vi "CreateSingleVibrationTDMSFile.vi"(0 "Requested Directory":path, 1 "Device":T4, 2 "Hierarchy":T1, 5 "Number of Channels":i32=18, 7 "Tach?":bool=TRUE, 9 "Pairs?":bool=TRUE, 11 "All Accelerometers?":bool=TRUE, 12 "sampling info":cluster{"Fs":dbl, "#s":dbl}={"Fs"=10000.0, "#s"=100000.0} {"Fs" format="%.2p"}, 13 "Running Speed (RPM)":dbl=3600.0, 14 "Amplitude":T11={"1x"=1.0, "2x"=0.5, "3x"=0.25, "8.5x"=1.0, "30x"=1.0}) -> (4 "Created File":path, 15 "error out":errorcluster)   [LabVIEW 2017]
uses:
  <vilib>/addons/InsightCM/MessageBus/Base/controls/Device.ctl
  <vilib>/addons/InsightCM/MessageBus/Base/controls/KeyValuePair.ctl
  <vilib>/addons/InsightCM/MessageBus/Base/controls/DeviceState.ctl
  <vilib>/addons/InsightCM/MessageBus/Base/controls/DataGroup.ctl
  <vilib>/addons/InsightCM/MessageBus/Base/controls/BurstModeTrigger.ctl
  <vilib>/addons/InsightCM/MessageBus/Base/controls/Trigger.ctl
  <vilib>/addons/InsightCM/MessageBus/Base/controls/Condition.ctl
  <vilib>/addons/InsightCM/Utilities/TDMSFileGenerator/controls/Hierarchy_All.ctl
  <vilib>/addons/InsightCM/Utilities/TDMSFileGenerator/controls/Hierarchy_Line.ctl
  <vilib>/addons/InsightCM/Utilities/TDMSFileGenerator/controls/Hierarchy_Equipment.ctl
  <vilib>/measure/NI_MABase.lvlib
  <vilib>/addons/Sound and Vibration/svt_DAQmx/Configuration XControl/Controls/svx_DAQ_RotationDirection.ctl
  <vilib>/addons/Sound and Vibration/svt_DAQmx/Configuration XControl/SVX NI-DAQmx AI Configuration XControl.xctl
  <vilib>/addons/Sound and Vibration/svt_DAQmx/Configuration XControl/Controls/svx_DAQ_Tach_Slope.ctl
panel:
  out "Array":i32[](array[numeric])
  out "Channel Names":string[](array[string])
  out "Waveforms":waveform(sgl)[](graph)
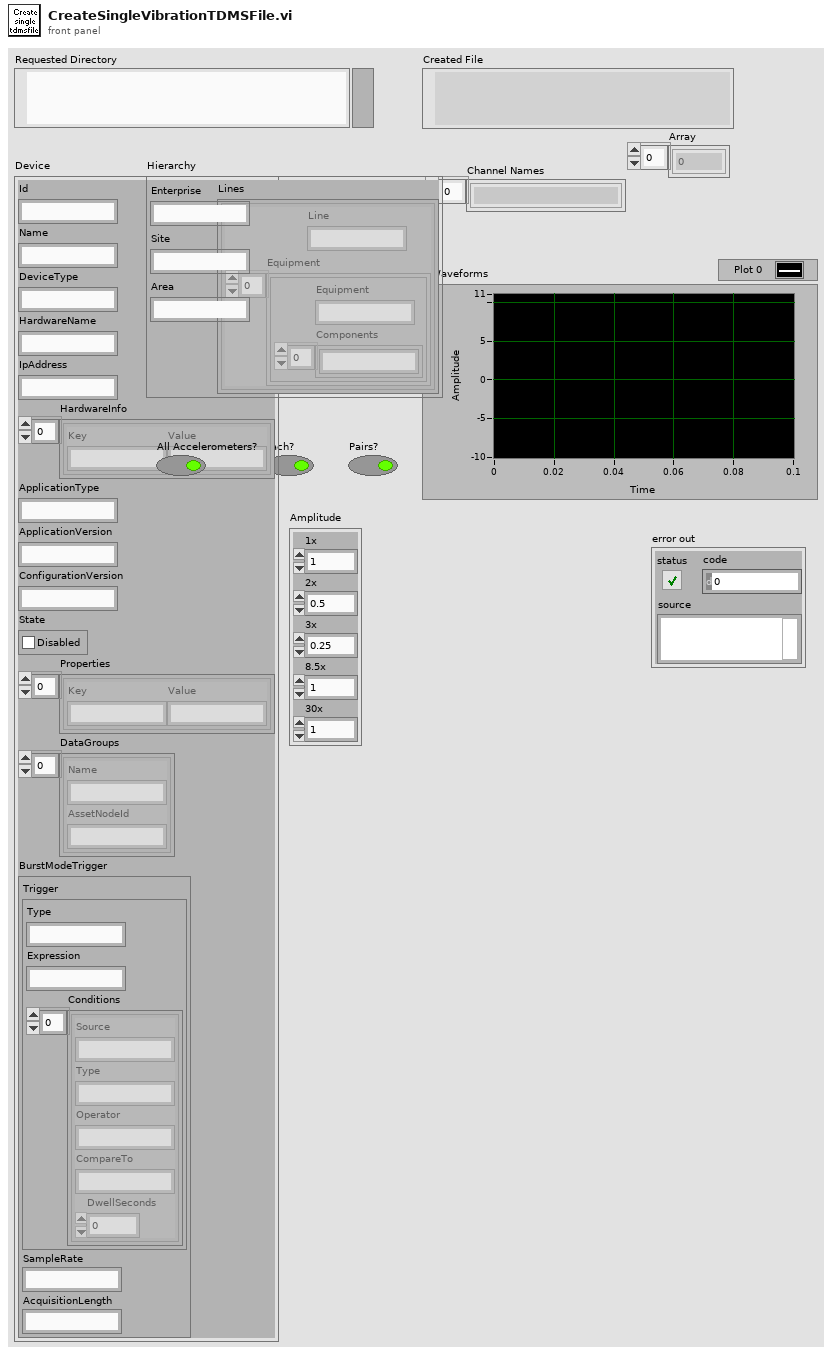
[diagram p1: front panel]
types:
  T1 = typedef "Hierarchy_All.ctl" = cluster{"Enterprise":string, "Site":string, "Area":string, "Lines":T2[]}
  T2 = typedef "Hierarchy_Line.ctl" = cluster{"Line":string, "Equipment":T3[]}
  T3 = typedef "Hierarchy_Equipment.ctl" = cluster{"Equipment":string, "Components":string[]}
  T4 = typedef "Device.ctl" = cluster{"Id":string, "Name":string, "DeviceType":string, "HardwareName":string, "IpAddress":string, "HardwareInfo":T5[], "ApplicationType":string, "ApplicationVersion":string, "ConfigurationVersion":string, "State":T6, "Properties":T5[], "DataGroups":T7[], "BurstModeTrigger":T8}
  T5 = typedef "KeyValuePair.ctl" = cluster{"Key":string, "Value":string}
  T6 = typedef "DeviceState.ctl" = cluster{"Disabled":bool}
  T7 = typedef "DataGroup.ctl" = cluster{"Name":string, "AssetNodeId":string}
  T8 = typedef "BurstModeTrigger.ctl" = cluster{"Trigger":T9, "SampleRate":string, "AcquisitionLength":string}
  T9 = typedef "Trigger.ctl" = cluster{"Type":string, "Expression":string, "Conditions":T10[]}
  T10 = typedef "Condition.ctl" = cluster{"Source":string, "Type":string, "Operator":string, "CompareTo":string, "DwellSeconds":dbl}
  T11 = cluster{"1x":dbl, "2x":dbl, "3x":dbl, "8.5x":dbl, "30x":dbl}
  T12 = enum16{"open", "open or create", "create or replace", "create", "open (read-only)"}
  T13 = typedef "SVX NI-DAQmx AI Configuration XControl.xctl/svx_DAQ_Tach_Slope.ctl" = enum16{"Rising", "Falling"}
  T14 = typedef "SVX NI-DAQmx AI Configuration XControl.xctl/svx_DAQ_RotationDirection.ctl" = enum16{"CW", "CCW"}
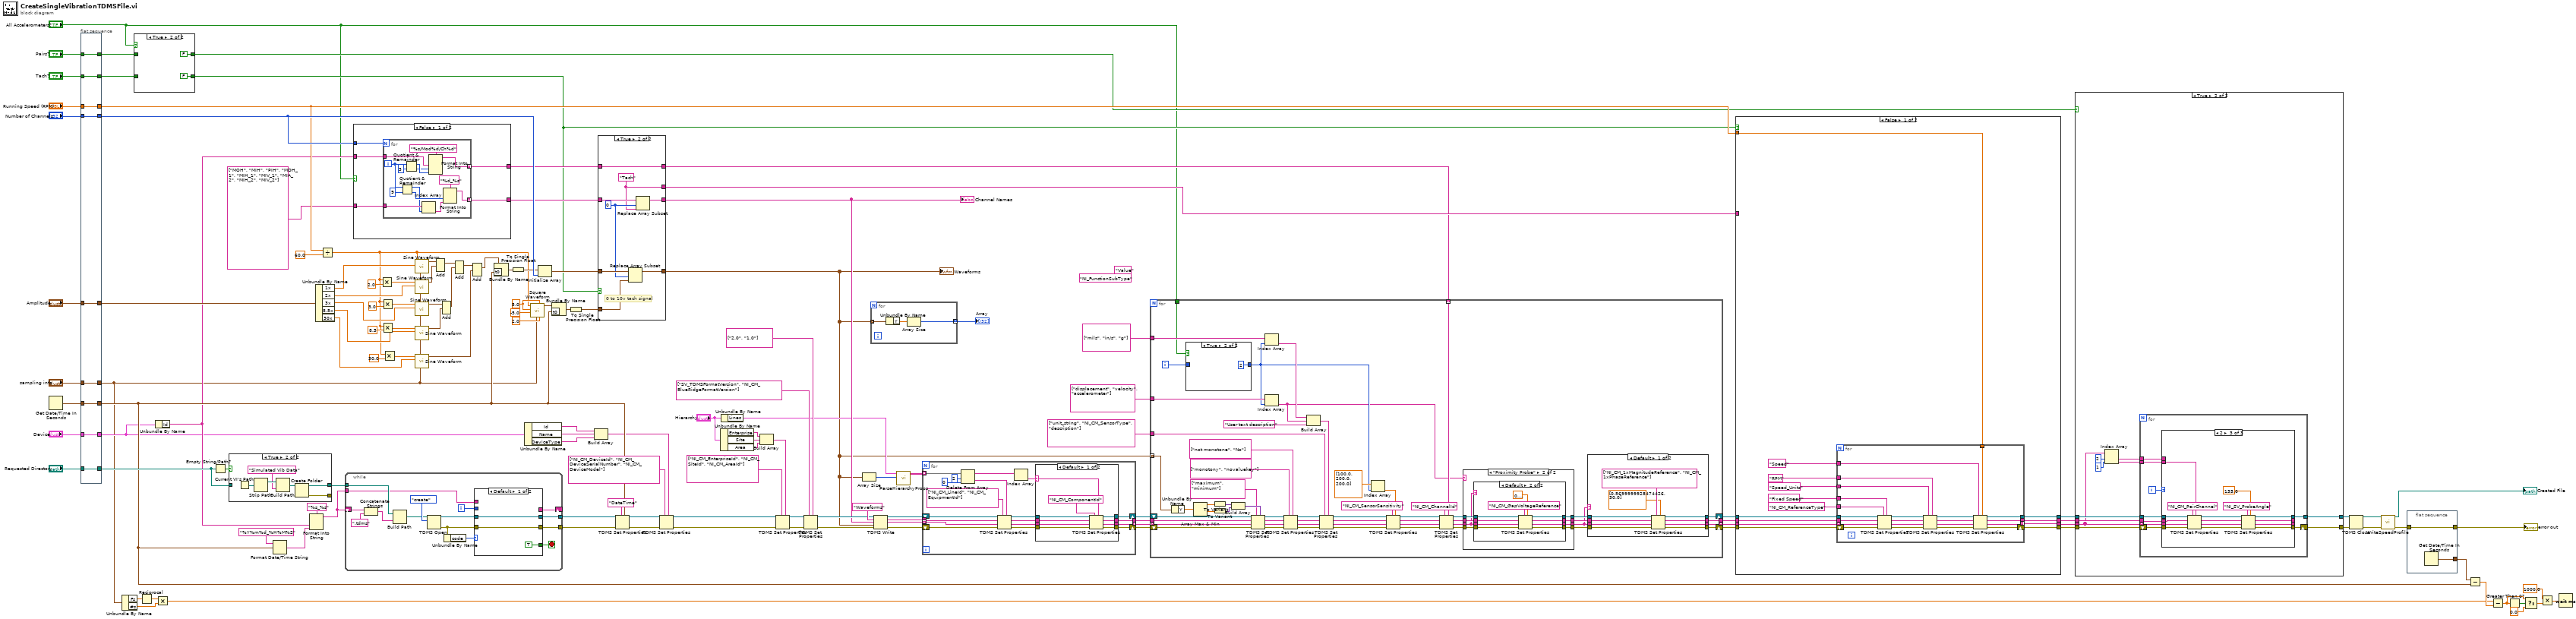
[diagram p0: block diagram]
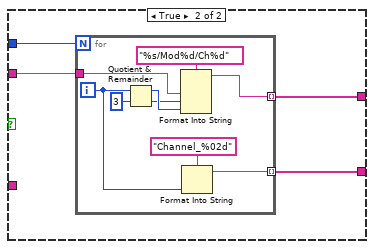
[diagram p2: hidden frame]
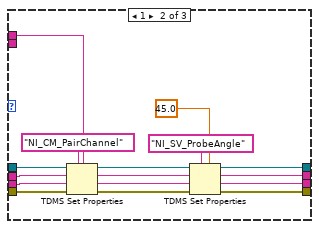
[diagram p7: hidden frame]
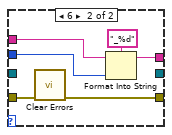
[diagram p8: hidden frame]
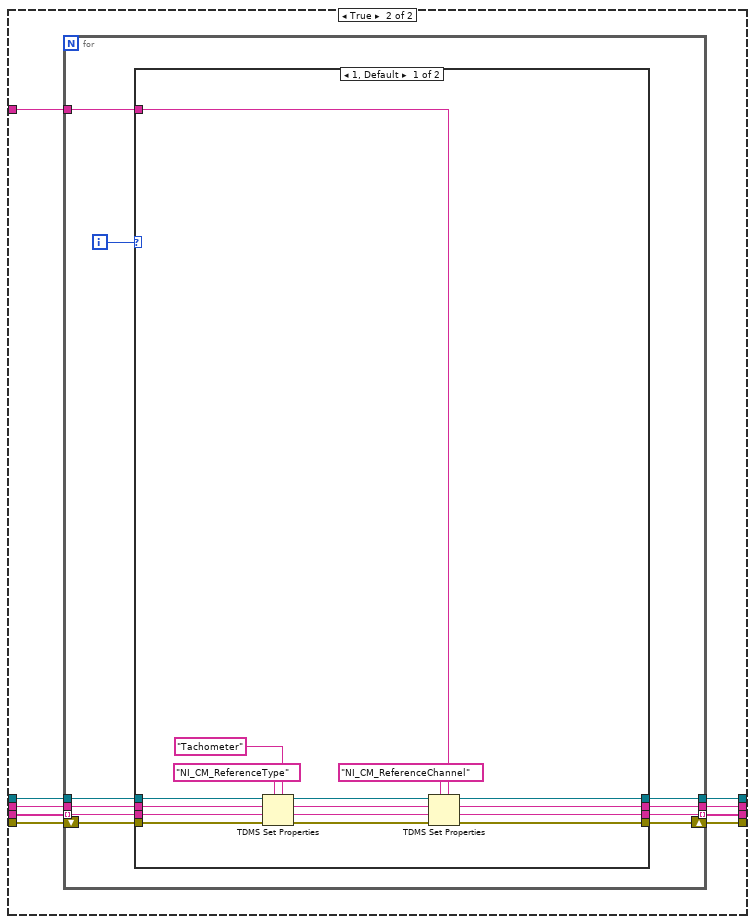
[diagram p10: hidden frame]
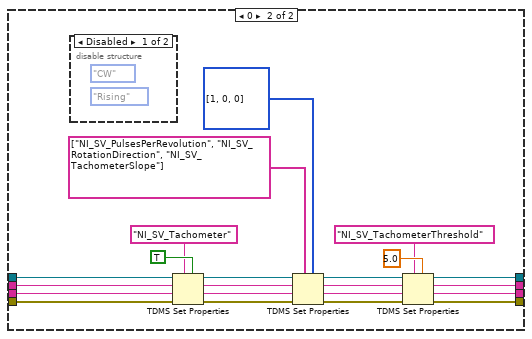
[diagram p11: hidden frame]
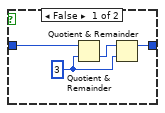
[diagram p13: hidden frame]
diagram:
  (unwired) "NI_FunctionSubType"
  w69 = 5.0 ("amplitude")
  (unwired) "Value"
  n1 = Get Date/Time In Seconds() -> (seconds since 1Jan1904=w92:timestamp)
  n2 = flat-sequence {
    tunnel: [w144] -> w101
    tunnel: "Requested Directory" -> [w144]
    tunnel: [w143] -> w11
    tunnel: "sampling info" -> [w143]
    tunnel: [w142] -> w98
    tunnel: "Amplitude" -> [w142]
    tunnel: [w141] -> w96
    tunnel: "Number of Channels" -> [w141]
    tunnel: [w140] -> w94
    tunnel: "Running Speed (RPM)" -> [w140]
    tunnel: [w139] -> w13
    tunnel: "Tach?" -> [w139]
    tunnel: [w138] -> w67
    tunnel: w92 -> [w138]
    tunnel: [w137] -> w15
    tunnel: "Pairs?" -> [w137]
    tunnel: "Device" -> [w136]
    tunnel: [w136] -> w43
    frame #0 {
    }
  }
  n3 = Unbundle By Name(w11) -> ("Fs"=w90:dbl, "#s"=w88:dbl)
  n4 = case shown="True" "All Accelerometers?" {
    tunnel: [w146 FALSE ("Pairs?")] -> w14
    tunnel: w15 -> [w146 _]
    tunnel: [w145 FALSE ("Tach?")] -> w12
    tunnel: w13 -> [w145 _]
    frame False {
    }
    frame True {
    }
  }
  n5 = Reciprocal(x=w90) -> (1/x=w89:dbl)
  n6 = Unbundle By Name(w43) -> ("Id"=w44:string)
  n7 = Multiply(x=w89, y=w88) -> (x*y=w86:dbl)
  n8 = Empty String/Path?(string/path=w101) -> (empty?=w121:bool)
  n9 = case shown="True" w121 {
    tunnel: [w149 w151] -> w122
    tunnel: w101 -> [w149 _]
    tunnel: [_ w150] -> _
    frame False {
    }
    frame True {
      n10 = Current VI's Path() -> (path=w155:path)
      n11 = Strip Path(path=w155) -> (stripped path=w154:path)  [unwired: 1 out]
      n12 = Build Path(base path=w154, name or relative path="Simulated Vib Data") -> (appended path=w152:path)
      n13 = Create Folder(path (use dialog)=w152) -> (created path=w151:path, error out=w150:errorcluster)  [unwired: 2 in, 1 out]
    }
  }
  n14 = Format Date/Time String(time format string (%c)="%Y%m%d_%H%M%S" ("format string"), seconds (now)=w67) -> (date/time string=w125:string)  [unwired: 1 in]
  n15 = Format Into String(format string="%s_%s", w44, w125) -> (resulting string=w103:string)  [unwired: 2 in, 1 out]
  n16 = Unbundle By Name(w98) -> ("1x"=w106:dbl, "2x"=w107:dbl, "3x"=w104:dbl, "8.5x"=w105:dbl, "30x"=w7:dbl)
  n17 = Divide(x=w94, y=60.0) -> (x/y=w8:dbl)
  n18 = while {
    tunnel: [w164] -> w132
    tunnel: [w166] -> w131
    tunnel: w122 -> [w168]
    shift-right: [w157] -> _
    shift-left: w103 -> [w161]
    tunnel: w103 -> [w159]
    i -> [w158]
    stop <- w167 stop-if-true
    n19 = Concatenate Strings(w161, ".tdms" ("format string")) -> (w160:string)
    n20 = Build Path(base path=w168, name or relative path=w160) -> (appended path=w169:path)
    n21 = TDMS Open(10:T12."create" ("operation (0:open)"), 11:w169) -> (0:w162:errorcluster, 3:w165:refnum<k34>)  [unwired: 5 in]
    n22 = Unbundle By Name(w162) -> ("code"=w163:i32)
    n23 = case shown="Default" w163 {
      tunnel: [TRUE _] -> w167
      tunnel: [w172 _] -> w166
      tunnel: w165 -> [w172 _]
      tunnel: [w171 w178] -> w164
      tunnel: w162 -> [w171 w179]
      tunnel: w159 -> [_ w177]
      tunnel: w158 -> [_ w175]
      tunnel: [_ w174] -> w157
      frame Default {
      }
      frame 6 {
        n24 = call <vilib>:"Clear Errors.vi"("error in (no error)"=w179) -> ("error out"=w178:errorcluster)  [unwired: 5 in, 1 out]
        n25 = Format Into String(format string="_%d", initial string=w177, w175) -> (resulting string=w174:string)  [unwired: 1 in, 1 out]
      }
    }
  }
  n26 = case shown="False" "All Accelerometers?" {
    tunnel: w96 -> [w184 w202]
    tunnel: string[] ["MOH", "MIH", "PIH", "MOH_1", "MIH_1", "MIV_1", "MIA_2", "MIH_2", "MIV_2"] ("property names") -> [w183 _]
    tunnel: [w182 w201] -> w60
    tunnel: [w181 w200] -> w59
    tunnel: w44 -> [w180 w199]
    frame False {
      n27 = for {
        N: w184 -> [_]
        tunnel: [w198] -> w181 mode=indexing
        tunnel: w180 -> [w197]
        tunnel: w183 -> [w187]
        tunnel: [w189] -> w182 mode=indexing
        i -> [w192]
        n28 = Quotient & Remainder(x=w192, y=9) -> (x-y*floor(x/y)=w185:i32, floor(x/y)=w188:i32)
        n29 = Quotient & Remainder(x=w192, y=3) -> (x-y*floor(x/y)=w195:i32, floor(x/y)=w194:i32)
        n30 = Index Array(array=w187, index=w185) -> (element=w186:string)
        n31 = Format Into String(format string="%s/Mod%d/Ch%d", w197, w194, w195) -> (resulting string=w198:string)  [unwired: 2 in, 1 out]
        n32 = Format Into String(format string="%d_%s", w188, w186) -> (resulting string=w189:string)  [unwired: 2 in, 1 out]
      }
    }
    frame True {
      n33 = for {
        N: w202 -> [_]
        tunnel: [w211] -> w200 mode=indexing
        tunnel: w199 -> [w210]
        tunnel: [w203] -> w201 mode=indexing
        i -> [w204]
        n34 = Quotient & Remainder(x=w204, y=3) -> (x-y*floor(x/y)=w208:i32, floor(x/y)=w207:i32)
        n35 = Format Into String(format string="%s/Mod%d/Ch%d", w210, w207, w208) -> (resulting string=w211:string)  [unwired: 2 in, 1 out]
        n36 = Format Into String(format string="Channel_%02d", w204) -> (resulting string=w203:string)  [unwired: 2 in, 1 out]
      }
    }
  }
  n37 = Multiply(x=w8, y=2.0) -> (x*y=w120:dbl)
  n38 = Multiply(x=w8, y=3.0) -> (x*y=w116:dbl)
  n39 = Multiply(x=w8, y=8.5) -> (x*y=w115:dbl)
  n40 = Multiply(x=w8, y=30.0) -> (x*y=w9:dbl)
  n41 = call <vilib>:"Sine Waveform.vi"("sampling info"=w11, "amplitude"=w106, "frequency"=w8) -> ("signal out"=w114:waveform(dbl))  [unwired: 7 in, 1 out]
  n42 = call <vilib>:"Sine Waveform.vi"("sampling info"=w11, "amplitude"=w107, "frequency"=w120) -> ("signal out"=w113:waveform(dbl))  [unwired: 7 in, 1 out]
  n43 = call <vilib>:"Sine Waveform.vi"("sampling info"=w11, "amplitude"=w104, "frequency"=w116) -> ("signal out"=w112:waveform(dbl))  [unwired: 7 in, 1 out]
  n44 = call <vilib>:"Sine Waveform.vi"("sampling info"=w11, "amplitude"=w105, "frequency"=w115) -> ("signal out"=w111:waveform(dbl))  [unwired: 7 in, 1 out]
  n45 = call <vilib>:"Sine Waveform.vi"("sampling info"=w11, "amplitude"=w7, "frequency"=w9) -> ("signal out"=w5:waveform(dbl))  [unwired: 7 in, 1 out]
  n46 = Add(1:w113, 2:w114) -> (0:w110:waveform(dbl))  [unwired: 1 in, 1 out]
  n47 = Add(1:w111, 2:w112) -> (0:w109:waveform(dbl))  [unwired: 1 in, 1 out]
  n48 = Add(1:w109, 2:w110) -> (0:w6:waveform(dbl))  [unwired: 1 in, 1 out]
  n49 = Add(1:w5, 2:w6) -> (0:w4:waveform(dbl))  [unwired: 1 in, 1 out]
  n50 = Bundle By Name(cluster=w4, "t0"=w67) -> (w73:waveform(dbl))
  n51 = To Single Precision Float(number=w73) -> (single precision float=w72:waveform(sgl))
  n52 = Unbundle By Name(w43) -> ("Id"=w41:string, "Name"=w42:string, "DeviceType"=w40:string)
  n53 = call <vilib>:"Square Waveform.vi"("duty cycle (%)"=2.0, "offset"=w69, "sampling info"=w11, "phase"=-5.0, "amplitude"=w69, "frequency"=w8) -> ("signal out"=w71:waveform(dbl))  [unwired: 4 in, 1 out]
  n54 = Initialize Array(w72, w96) -> (w108:waveform(sgl)[])
  n55 = Bundle By Name(cluster=w71, "t0"=w67) -> (w66:waveform(dbl))
  n56 = To Single Precision Float(number=w66) -> (single precision float=w65:waveform(sgl))
  n57 = Build Array(w41, w42, w40) -> (w39:string[])
  n58 = case shown="True" w12 {
    tunnel: w108 -> [w214 w222]
    tunnel: [w214 w221] -> w2
    tunnel: w60 -> [w213 w219]
    tunnel: w65 -> [_ w220]
    tunnel: [w213 w218] -> w58
    tunnel: w59 -> [w212 w216]
    tunnel: [w212 w216] -> w56
    tunnel: [_ w215] -> w57
    frame False {
    }
    frame True {
      w215 = "Tach" ("new element/subarray")
      w217 = 0 ("index")
      # "0 to 10v tach signal"
      n59 = Replace Array Subset(array=w222, new element=w220, index=w217) -> (w221:waveform(sgl)[])
      n60 = Replace Array Subset(array=w219, new element=w215, index=w217) -> (w218:string[])
    }
  }
  "Waveforms" <- w2
  "Channel Names" <- w58
  n61 = TDMS Set Properties(5:w67, 7:"DateTime" ("property names"), 8:w132, 11:w131) -> (0:w128:errorcluster, 3:w127:refnum<k34>)  [unwired: 2 in, 2 out]
  n62 = TDMS Set Properties(5:w39, 7:string[] ["NI_CM_DeviceId", "NI_CM_DeviceSerialNumber", "NI_CM_DeviceModel"], 8:w128, 11:w127) -> (0:w37:errorcluster, 3:w38:refnum<k34>)  [unwired: 2 in, 2 out]
  n63 = Unbundle By Name("Hierarchy") -> ("Enterprise"=w32:string, "Site"=w33:string, "Area"=w31:string)
  n64 = Unbundle By Name("Hierarchy") -> ("Lines"=w28:T2[])
  n65 = Build Array(w32, w33, w31) -> (w30:string[])
  n66 = TDMS Set Properties(5:w30, 7:string[] ["NI_CM_EnterpriseId", "NI_CM_SiteId", "NI_CM_AreaId"], 8:w37, 11:w38) -> (0:w36:errorcluster, 3:w35:refnum<k34>)  [unwired: 2 in, 2 out]
  n67 = TDMS Set Properties(5:string[] ["2.0", "1.0"] ("property names"), 7:string[] ["SV_TDMSFormatVersion", "NI_CM_BlueRidgeFormatVersion"] ("property names"), 8:w36, 11:w35) -> (0:w75:errorcluster, 3:w76:refnum<k34>)  [unwired: 2 in, 2 out]
  n68 = Array Size(array=w2) -> (size(s)=w21:i32)
  n69 = for {
    tunnel: w2 -> [w225] mode=indexing
    tunnel: [w223] -> w1 mode=indexing
    n70 = Unbundle By Name(w225) -> ("Y"=w224:sgl[])
    n71 = Array Size(array=w224) -> (size(s)=w223:i32)
  }
  "Array" <- w1
  n72 = TDMS Write(0:w76, 5:"Waveforms" ("group name in (Untitled)"), 7:w58, 9:w2, 11:w75) -> (4:w24:refnum<k34>, 6:w23:string, 8:w22:string[], 15:w25:errorcluster)  [unwired: 1 in]
  n73 = call <vilib>:"ParseHierarchyProps.vi"("Number of Channels"=w21, "Lines"=w28) -> ("Array of Hierarchy Properties"=w26:string[][])  [unwired: 9 in]
  n74 = for {
    tunnel: w26 -> [w240] mode=indexing
    shift-right: [w233] -> w19
    shift-left: w25 -> [w243]
    shift-right: [w232] -> w20
    shift-left: w24 -> [w244]
    tunnel: w23 -> [w241]
    tunnel: w22 -> [w242] mode=indexing
    tunnel: [w228] -> w18
    tunnel: [w227] -> w17 mode=indexing
    n75 = Delete From Array(array=w240, length=2, index=0) -> (deleted portion=w238:string[], array with subset deleted=w236:string[])
    n76 = TDMS Set Properties(5:w238, 7:string[] ["NI_CM_LineId", "NI_CM_EquipmentId"], 8:w243, 9:w242, 10:w241, 11:w244) -> (0:w234:errorcluster, 1:w229:string, 2:w230:string, 3:w231:refnum<k34>)
    n77 = Index Array(array=w236) -> (element=w235:string)  [unwired: 1 in]
    n78 = case shown="Default" w235 {
      selector: w235 -> [w248 _]
      tunnel: w234 -> [w254 w258]
      tunnel: [w253 w258] -> w233
      tunnel: [w251 w257] -> w232
      tunnel: w231 -> [w252 w257]
      tunnel: w230 -> [w250 w256]
      tunnel: w229 -> [w249 w255]
      tunnel: [w246 w256] -> w228
      tunnel: [w245 w255] -> w227
      frame Default {
        n79 = TDMS Set Properties(5:w248, 7:"NI_CM_ComponentId" ("property names"), 8:w254, 9:w249, 10:w250, 11:w252) -> (0:w253:errorcluster, 1:w245:string, 2:w246:string, 3:w251:refnum<k34>)
      }
      frame "" {
      }
    }
  }
  n80 = for {
    tunnel: w18 -> [w272]
    tunnel: w17 -> [w273] mode=indexing
    shift-right: [w288] -> w124
    shift-left: w19 -> [w274]
    tunnel: string[] ["unit_string", "NI_CM_SensorType", "description"] ("property names") -> [w315]
    tunnel: [w290] -> w123
    tunnel: string[] ["mils", "in/s", "g"] -> [w313]
    tunnel: string[] ["displacement", "velocity", "accelerometer"] -> [w311]
    tunnel: [w289] -> w62 mode=indexing
    tunnel: w56 -> [w300] mode=indexing
    tunnel: w2 -> [w270] mode=indexing
    shift-right: [w260] -> w27
    shift-left: w20 -> [w271]
    tunnel: "All Accelerometers?" -> [w259]
    i -> [w296]
    n81 = Unbundle By Name(w270) -> ("Y"=w275:sgl[])
    n82 = case shown="True" w259 {
      tunnel: [w317 2] -> w304
      tunnel: w296 -> [w316 _]
      frame False {
        w318 = 3 ("y")
        n83 = Quotient & Remainder(x=w316, y=w318) -> (floor(x/y)=w319:i32)  [unwired: 1 out]
        n84 = Quotient & Remainder(x=w319, y=w318) -> (x-y*floor(x/y)=w317:i32)  [unwired: 1 out]
      }
      frame True {
      }
    }
    n85 = Array Max & Min(array=w275) -> (max value=w277:sgl, min value=w278:sgl)  [unwired: 2 out]
    n86 = To Variant(anything=w277) -> (Variant=w279:variant)
    n87 = To Variant(anything=w278) -> (Variant=w280:variant)
    n88 = Build Array(w279, w280) -> (w281:variant[])
    n89 = TDMS Set Properties(5:w281, 7:string[] ["maximum", "minimum"] ("property names"), 8:w274, 9:w273, 10:w272, 11:w271) -> (0:w282:errorcluster, 1:w285:string, 2:w283:string, 3:w284:refnum<k34>)
    n90 = Index Array(array=w313, index=w304) -> (element=w312:string)
    n91 = Index Array(array=w311, index=w304) -> (element=w295:string)
    n92 = TDMS Set Properties(5:string[] ["not monotone", "No"] ("property names"), 7:string[] ["monotony", "novaluekey"] ("property names"), 8:w282, 9:w285, 10:w283, 11:w284) -> (0:w266:errorcluster, 1:w267:string, 2:w268:string, 3:w269:refnum<k34>)
    n93 = Build Array(w312, w295, "User text description") -> (w314:string[])
    n94 = TDMS Set Properties(5:w314, 7:w315, 8:w266, 9:w267, 10:w268, 11:w269) -> (0:w310:errorcluster, 1:w307:string, 2:w308:string, 3:w309:refnum<k34>)
    n95 = Index Array(array=sgl[] [100.0, 200.0, 200.0], index=w304) -> (element=w303:sgl)
    n96 = TDMS Set Properties(5:w303, 7:"NI_CM_SensorSensitivity", 8:w310, 9:w307, 10:w308, 11:w309) -> (0:w302:errorcluster, 1:w297:string, 2:w298:string, 3:w299:refnum<k34>)
    n97 = TDMS Set Properties(5:w300, 7:"NI_CM_ChannelId", 8:w302, 9:w297, 10:w298, 11:w299) -> (0:w262:errorcluster, 1:w263:string, 2:w264:string, 3:w265:refnum<k34>)
    n98 = case shown="\"Proximity Probe\"" w295 {
      tunnel: [w338 w345] -> w293
      tunnel: w262 -> [w338 w346]
      tunnel: w265 -> [w337 w344]
      tunnel: w264 -> [w336 w343]
      tunnel: w263 -> [w335 w339]
      tunnel: [w337 w342] -> w294
      tunnel: [w336 w341] -> w292
      tunnel: [w335 w340] -> w291
      frame Default {
      }
      frame "Proximity Probe" {
        n99 = case shown="Default" w339 {
          tunnel: w346 -> [w347 w360]
          tunnel: [w347 w359] -> w345
          tunnel: w344 -> [w350 w357]
          tunnel: w343 -> [w349 w356]
          tunnel: w339 -> [w348 w355]
          tunnel: [w350 w354] -> w342
          tunnel: [w349 w353] -> w341
          tunnel: [w348 w352] -> w340
          frame "Tach" {
          }
          frame Default {
            n100 = TDMS Set Properties(5:sgl 0.1, 7:"NI_CM_GapVoltageReference", 8:w360, 9:w355, 10:w356, 11:w357) -> (0:w359:errorcluster, 1:w352:string, 2:w353:string, 3:w354:refnum<k34>)
          }
        }
      }
    }
    n101 = case shown="Default" w291 {
      tunnel: [w329 w334] -> w288
      tunnel: w293 -> [w330 w334]
      tunnel: w294 -> [w328 w333]
      tunnel: w292 -> [w327 w332]
      tunnel: w291 -> [w326 w331]
      tunnel: [w325 w333] -> w260
      tunnel: [w324 w332] -> w290
      tunnel: [w323 w331] -> w289
      frame Default {
        n102 = TDMS Set Properties(5:sgl[] [0.57, 30.0], 7:string[] ["NI_CM_1xMagnitudeReference", "NI_CM_1xPhaseReference"] ("property names"), 8:w330, 9:w326, 10:w327, 11:w328) -> (0:w329:errorcluster, 1:w323:string, 2:w324:string, 3:w325:refnum<k34>)
      }
      frame "Tach" {
      }
    }
  }
  n103 = case shown="False" w12 {
    tunnel: w123 -> [w373 w403]
    tunnel: [w366 w399] -> w53
    tunnel: w124 -> [w372 w405]
    tunnel: [w367 w397] -> w55
    tunnel: [w365 w400] -> w52
    tunnel: w27 -> [w374 w404]
    tunnel: w94 -> [w368 _]
    tunnel: w62 -> [w364 w402]
    tunnel: w57 -> [_ w401]
    tunnel: [w361 w398] -> w54
    frame False {
      n104 = for {
        tunnel: w373 -> [w381]
        tunnel: w364 -> [w382] mode=indexing
        shift-right: [w390] -> w367
        shift-left: w372 -> [w385]
        tunnel: w374 -> [w378]
        tunnel: "Speed_Units" -> [w396]
        tunnel: "RPM" -> [w395]
        tunnel: "Speed" -> [w389]
        tunnel: w368 -> [w388]
        tunnel: [w387] -> w366
        tunnel: [w386] -> w365
        tunnel: "Fixed Speed" -> [w377]
        tunnel: "NI_CM_ReferenceType" -> [w376]
        tunnel: [w375] -> w361 mode=indexing
        n105 = TDMS Set Properties(5:w377, 7:w376, 8:w385, 9:w382, 10:w381, 11:w378) -> (0:w384:errorcluster, 1:w383:string, 2:w380:string, 3:w379:refnum<k34>)
        n106 = TDMS Set Properties(5:w395, 7:w396, 8:w384, 9:w383, 10:w380, 11:w379) -> (0:w391:errorcluster, 1:w392:string, 2:w393:string, 3:w394:refnum<k34>)
        n107 = TDMS Set Properties(5:w388, 7:w389, 8:w391, 9:w392, 10:w393, 11:w394) -> (0:w390:errorcluster, 1:w375:string, 2:w387:string, 3:w386:refnum<k34>)
      }
    }
    frame True {
      n108 = for {
        tunnel: w402 -> [w413] mode=indexing
        shift-right: [w414] -> w397
        shift-left: w405 -> [w415]
        tunnel: w404 -> [w412]
        tunnel: [w411] -> w400
        tunnel: w403 -> [w410]
        tunnel: [w409] -> w399
        tunnel: w401 -> [w408]
        tunnel: [w407] -> w398 mode=indexing
        i -> [w406]
        n109 = case shown="1, Default" w406 {
          tunnel: w415 -> [w431 w438]
          tunnel: [w416 w433] -> w414
          tunnel: w413 -> [w430 w437]
          tunnel: w412 -> [w429 w439]
          tunnel: [w419 w435] -> w411
          tunnel: w410 -> [w428 w436]
          tunnel: [w418 w434] -> w409
          tunnel: w408 -> [w420 _]
          tunnel: [w417 w432] -> w407
          frame 1, Default {
            n110 = TDMS Set Properties(5:"Tachometer", 7:"NI_CM_ReferenceType", 8:w431, 9:w430, 10:w428, 11:w429) -> (0:w422:errorcluster, 1:w423:string, 2:w424:string, 3:w425:refnum<k34>)
            n111 = TDMS Set Properties(5:w420, 7:"NI_CM_ReferenceChannel", 8:w422, 9:w423, 10:w424, 11:w425) -> (0:w416:errorcluster, 1:w417:string, 2:w418:string, 3:w419:refnum<k34>)
          }
          frame 0 {
            n112 = disable-structure shown="Disabled" {
              frame Disabled {
                (unwired) svx_DAQ_Tach_Slope."Rising" ("Tach Slope")
                (unwired) svx_DAQ_RotationDirection."CW" ("Tach Direction")
              }
              frame Enabled {
              }
            }
            n113 = TDMS Set Properties(5:TRUE, 7:"NI_SV_Tachometer", 8:w438, 9:w437, 10:w436, 11:w439) -> (0:w445:errorcluster, 1:w444:string, 2:w443:string, 3:w442:refnum<k34>)
            n114 = TDMS Set Properties(5:i32[] [1, 0, 0], 7:string[] ["NI_SV_PulsesPerRevolution", "NI_SV_RotationDirection", "NI_SV_TachometerSlope"] ("property names"), 8:w445, 9:w444, 10:w443, 11:w442) -> (0:w451:errorcluster, 1:w450:string, 2:w449:string, 3:w448:refnum<k34>)
            n115 = TDMS Set Properties(5:sgl 5.0 ("amplitude"), 7:"NI_SV_TachometerThreshold", 8:w451, 9:w450, 10:w449, 11:w448) -> (0:w433:errorcluster, 1:w432:string, 2:w434:string, 3:w435:refnum<k34>)
          }
        }
      }
    }
  }
  n116 = case shown="True" w14 {
    tunnel: w55 -> [w454 w465]
    tunnel: w54 -> [_ w460]
    tunnel: w53 -> [_ w464]
    tunnel: w52 -> [w455 w463]
    tunnel: [w454 w457] -> w51
    tunnel: [w455 w456] -> w50
    frame False {
    }
    frame True {
      n117 = Index Array(array=w460, index #1=2 ("index"), index #2=1 ("index")) -> (element #1=w459:string, element #2=w458:string)
      n118 = for {
        tunnel: w460 -> [w471] mode=indexing
        tunnel: w464 -> [w472]
        tunnel: w463 -> [w473]
        shift-right: [w469] -> w457
        shift-left: w465 -> [w470]
        tunnel: [w468] -> w456
        tunnel: w459 -> [w467]
        tunnel: w458 -> [w466]
        i -> [w474]
        n119 = case shown="2" w474 {
          tunnel: w473 -> [w478 w490 w506]
          tunnel: w472 -> [w477 w487 w503]
          tunnel: w471 -> [w476 w486 w502]
          tunnel: w470 -> [w475 w483 w499]
          tunnel: [w475 w494 w510] -> w469
          tunnel: [w476 w493 w509] -> _
          tunnel: [w477 w492 w508] -> _
          tunnel: [w478 w491 w507] -> w468
          tunnel: w467 -> [_ w480 _]
          tunnel: w466 -> [_ _ w496]
          frame Default {
          }
          frame 1 {
            n120 = TDMS Set Properties(5:w480, 7:"NI_CM_PairChannel", 8:w483, 9:w486, 10:w487, 11:w490) -> (0:w484:errorcluster, 1:w485:string, 2:w488:string, 3:w489:refnum<k34>)
            n121 = TDMS Set Properties(5:sgl 45.0 ("amplitude"), 7:"NI_SV_ProbeAngle", 8:w484, 9:w485, 10:w488, 11:w489) -> (0:w494:errorcluster, 1:w493:string, 2:w492:string, 3:w491:refnum<k34>)
          }
          frame 2 {
            n122 = TDMS Set Properties(5:w496, 7:"NI_CM_PairChannel", 8:w499, 9:w502, 10:w503, 11:w506) -> (0:w500:errorcluster, 1:w501:string, 2:w504:string, 3:w505:refnum<k34>)
            n123 = TDMS Set Properties(5:sgl 135.0 ("amplitude"), 7:"NI_SV_ProbeAngle", 8:w500, 9:w501, 10:w504, 11:w505) -> (0:w510:errorcluster, 1:w509:string, 2:w508:string, 3:w507:refnum<k34>)
          }
        }
      }
    }
  }
  n124 = TDMS Close(8:w51, 11:w50) -> (0:w48:errorcluster, 3:w49:path)
  n125 = call <vilib>:"WriteSpeedProfile.vi"("error in (no error)"=w48, "TDMS File"=w49) -> ("error out"=w47:errorcluster, "TDMS File Out"=→"Created File":path)  [unwired: 8 in]
  n126 = flat-sequence {
    tunnel: [w512] -> w91
    tunnel: w47 -> [w512]
    tunnel: [w511] -> w85
    frame #0 {
      n127 = Get Date/Time In Seconds() -> (seconds since 1Jan1904=w511:timestamp)
    }
  }
  n128 = Subtract(x=w85, y=w67) -> (x-y=w87:dbl)
  n129 = Subtract(x=w86, y=w87) -> (x-y=w83:dbl)
  n130 = Greater Than 0?(x=w83) -> (x > 0?=w84:bool)
  n131 = Select(t=w83, s=w84, f=0.0) -> (s? t:f=w81:dbl)
  n132 = Multiply(x=1000.0, y=w81) -> (x*y=w79:dbl)
  n133 = Wait (ms)(milliseconds to wait=w79) -> ()  [unwired: 1 out]
  "error out" <- w91
